vi "RT_Read_Count_FIFO.vi"(6 "rt fifo":refnum<k33>, 8 "error in (no error)":errorcluster, 10 "Elements to read":u32) -> (0 "error out":errorcluster, 1 "Data":i32[](array[numeric]), 2 "# elements 2":u32, 3 "timed out?":bool)   [LabVIEW 2020]
uses:
  <vilib>/FPGAPlugInAG/cRIO-9040/niLvFpga_Open_cRIO-9040.vi
  <vilib>/Utility/error.llb/Error Cluster From Error Code.vi
  <vilib>/rvi/errors/niLvFpgaAdjustHostInterfaceError.vi
  <vilib>/rvi/interface/nirviOpenFPGA/nirviOpenFPGA.xnode
  FPGA Bitfiles/depapp_FPGATarget_FPGAmain_WC8wSYHNwdY.lvbitx
  FPGA_main.vi
  <vilib>/rvi/interface/nirviMethod/nirviMethod.xnode
  <vilib>/rvi/errors/niLvFpgaMergeErrorWithErrorCode.vi
  <vilib>/FPGAPlugInAG/cRIO-9040/niLvFpga_ReadFifo_cRIO-9040.vi
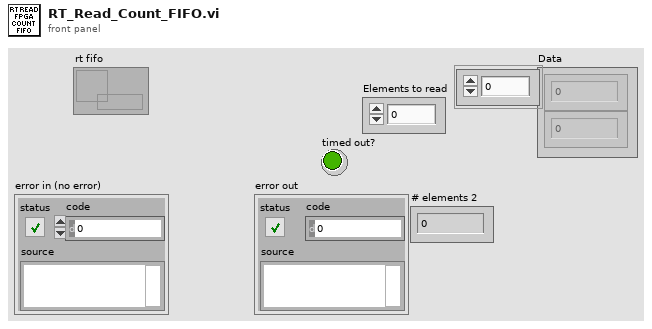
[diagram p1: front panel]
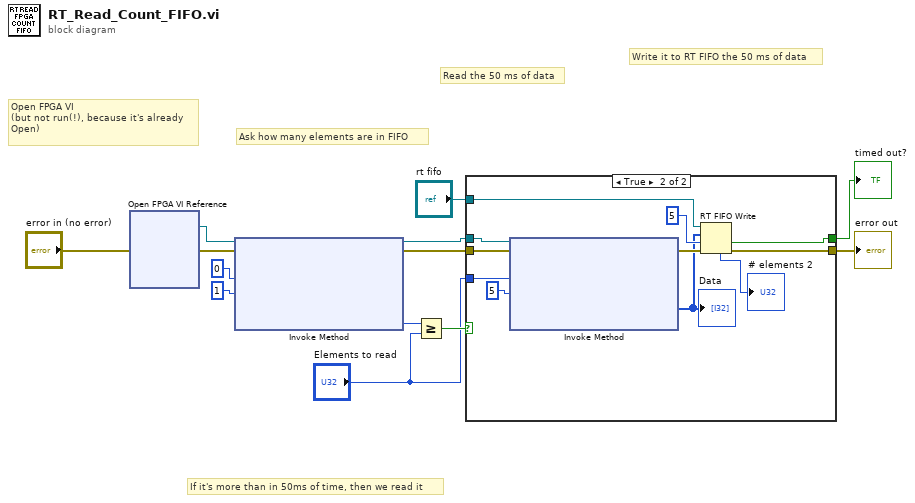
[diagram p0: block diagram]
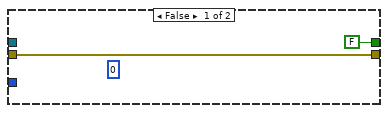
[diagram p2: hidden frame]
diagram:
  # "Write it to RT FIFO the 50 ms of data"
  # "Read the 50 ms of data"
  # "If it's more than in 50ms of time, then we read it"
  # "Ask how many elements are in FIFO"
  # "Open FPGA VI \n(but not run(!), because it's already \nOpen)"
  n1 = xnode "Open FPGA VI Reference"("error in"="error in (no error)") -> ("FPGA VI Reference Out"=w1:refnum<k20>, "error out"=w2:errorcluster)  [unwired: 1 in]
  n2 = xnode "Invoke Method"("FPGA VI Reference In"=w1, "error in"=w2, "Number of Elements"=u32 0, "Timeout (ms)"=1) -> ("FPGA VI Reference Out"=w10:refnum<k20>, "error out"=w11:errorcluster, "Elements Remaining"=w9:u32)  [unwired: 1 out]
  n3 = Greater Or Equal?(x=w9, y="Elements to read") -> (x >= y?=w6:bool)
  n4 = case shown="True" w6 {
    tunnel: w11 -> [w15 w25]
    tunnel: w10 -> [_ w24]
    tunnel: "rt fifo" -> [_ w23]
    tunnel: [w15 w20] -> w7
    tunnel: "Elements to read" -> [_ w19]
    tunnel: [FALSE ("timed out?") w18] -> w4
    frame False {
      (unwired) u32 0 ("# elements")
    }
    frame True {
      n5 = xnode "Invoke Method"("FPGA VI Reference In"=w24, "error in"=w25, "Number of Elements"=w19, "Timeout (ms)"=5) -> ("error out"=w21:errorcluster, "Data"=w16:i32[])  [unwired: 2 out]
      "Data" <- w16
      n6 = RT FIFO Write(0:w23, 1:w16, 2:5 ("timeout in ms (0)"), 3:w21) -> (7:→"# elements 2":u32, 10:w18:bool, 11:w20:errorcluster)  [unwired: 1 in, 1 out]
    }
  }
  "error out" <- w7
  "timed out?" <- w4
